vi "AutoBalance.vi"() -> (3 "Output Speed":dbl)   [LabVIEW 2011]
panel:
  in  "Initial Speed":dbl
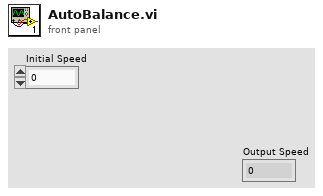
[diagram p1: front panel]
types:
  T1 = typedef "WPI_GyroDevRef.ctl" = cluster{"DevStatus":errorcluster, "Analog Module":T2, "Analog Channel":T3, "Offset":dbl, "Gain (VoltsPerDegree/Second)":dbl}
  T2 = typedef "FPGA_TypedefAnalogModule.ctl" = enum16{"Analog Module 1", "Analog Module 2"}
  T3 = typedef "FPGA_AIChannel.ctl" = enum8{"AI 1", "AI 2", "AI 3", "AI 4", "AI 5", "AI 6", "AI 7", "AI 8", "Invalid"}
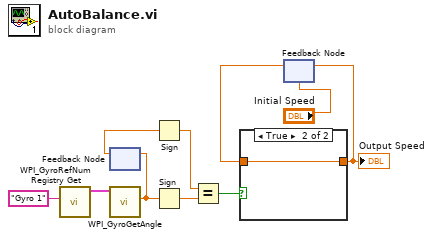
[diagram p0: block diagram]
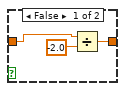
[diagram p2: hidden frame]
diagram:
  n1 = call <vilib>:"WPI_GyroRefNum Registry Get.vi"("refnum name"="Gyro 1") -> ("GyroDevRef"=w9:T1)  [unwired: 9 in, 1 out]
  n2 = feedback #1() -> (w5:dbl)  [unwired: 1 in]
  n3 = call <vilib>:"WPI_GyroGetAngle.vi"("GyroDevRef"=w9) -> ("Angle"=w4:dbl)  [unwired: 7 in, 3 out]
  n4 = feedback-in #1(w4) -> ()
  n5 = Sign(1:w5) -> (0:w8:dbl)
  n6 = Sign(1:w4) -> (0:w7:dbl)
  n7 = Equal?(x=w8, y=w7) -> (x = y?=w6:bool)
  n8 = feedback #2("Initial Speed") -> (w2:dbl)
  n9 = case shown="True" w6 {
    tunnel: w2 -> [w12 w14]
    tunnel: [w11 w14] -> w1
    frame False {
      n10 = Divide(x=w12, y=-2.0) -> (x/y=w11:dbl)
    }
    frame True {
    }
  }
  "Output Speed" <- w1
  n11 = feedback-in #2(w1) -> ()
